vi "setNotificationSettings.vi"(8 "error in (no error)":errorcluster, 10 "not_settings":bool[](array[boolean]), 11 "reference in":refnum<class "File Controller.lvclass">) -> (0 "error out":errorcluster, 3 "reference out":refnum<class "File Controller.lvclass">)   [LabVIEW 2014, in "File Controller.lvclass"]
uses:
  File Controller.lvclass
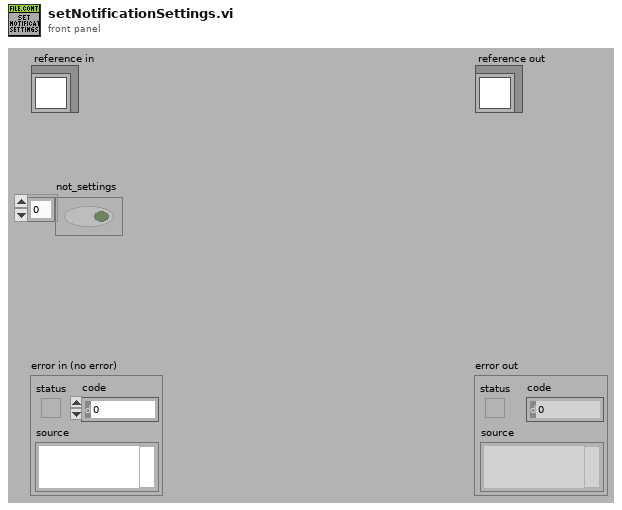
[diagram p1: front panel]
types:
  T1 = typedef "File Controller.lvclass/ObjectAttributesRef.ctl" = refnum<data-value>
  T2 = typedef "File Controller.lvclass/ObjectAttributes.ctl" = cluster{"MyAttribute":dbl, "excelFile_refs":refnum<class "excelFile.lvclass">[], "filePaths":path[], "outlookTemplatePaths":path[], "attachmentTemplatePaths":path[], "configFilePath":path, "not_setting":bool[], "python_ref":refnum<class "python.lvclass">}
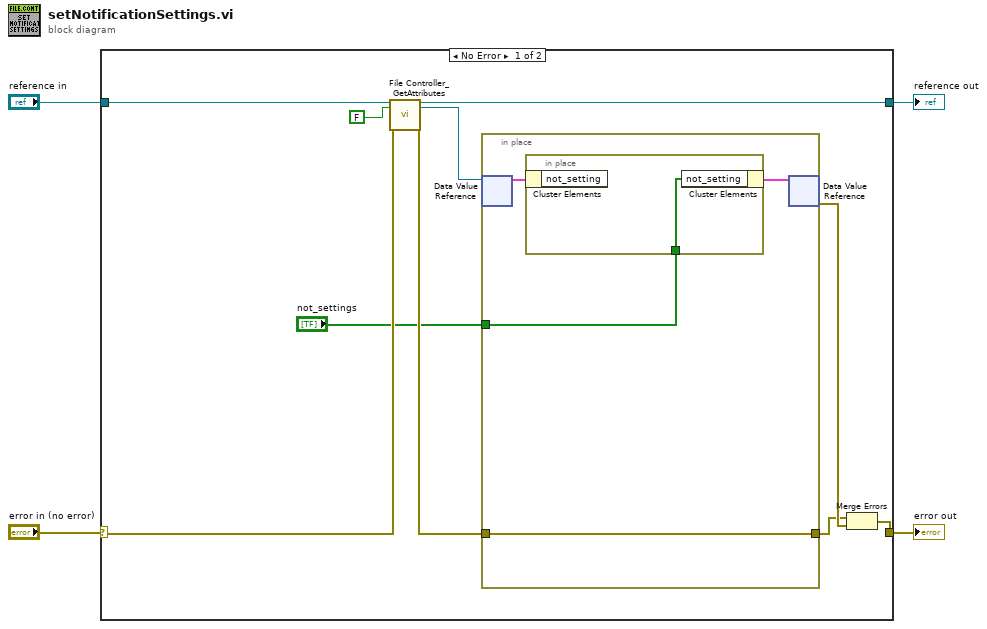
[diagram p0: block diagram]
diagram:
  n1 = case shown="No Error" "error in (no error)" {
    selector: "error in (no error)" -> [w9 w21]
    tunnel: [w14 w21] -> w3
    tunnel: [w7 w20] -> w1
    tunnel: "reference in" -> [w11 w20]
    frame No Error {
      n2 = call "File Controller_GetAttributes.vi"("reference in"=w11, "return data? (T)"=FALSE, "error in (no error)"=w9) -> ("reference out"=w7:refnum<class "File Controller.lvclass">, "attributes ref"=w6:T1, "error out"=w8:errorcluster)  [unwired: 13 in, 1 out]
      n3 = in-place {
        in-place-border: w8 -> [w16]
        in-place-border: [w16] -> w12
        in-place-border: "not_settings" -> [w15]
        n4 = in-place-dvr #1(w6) -> (w17:T2)  [unwired: 1 out]
        n5 = in-place {
          in-place-border: w15 -> [w19]
          n6 = in-place-cluster #2(w17) -> ()  [unwired: 1 out]
          n7 = in-place-cluster #2("not_setting"=w19) -> (w18:T2)
        }
        n8 = in-place-dvr #1(w18) -> (w13:errorcluster)  [unwired: 1 out]
      }
      n9 = Merge Errors(w12, w13) -> (w14:errorcluster)
    }
    frame Error {
    }
  }
  "error out" <- w3
  "reference out" <- w1
